vi "OG_HTML_String.vi"(11 "Cluster":T1) -> (3 "String":string)   [LabVIEW 2018]
uses:
  MainFrame/TypeDefs/InternalDataCluster.ctl
  Private Controls/Report Data Cluster.ctl
  Private Controls/Data Raw.ctl
  Data Operations.lvlib
  MainFrame/MainFrameLib.lvlib
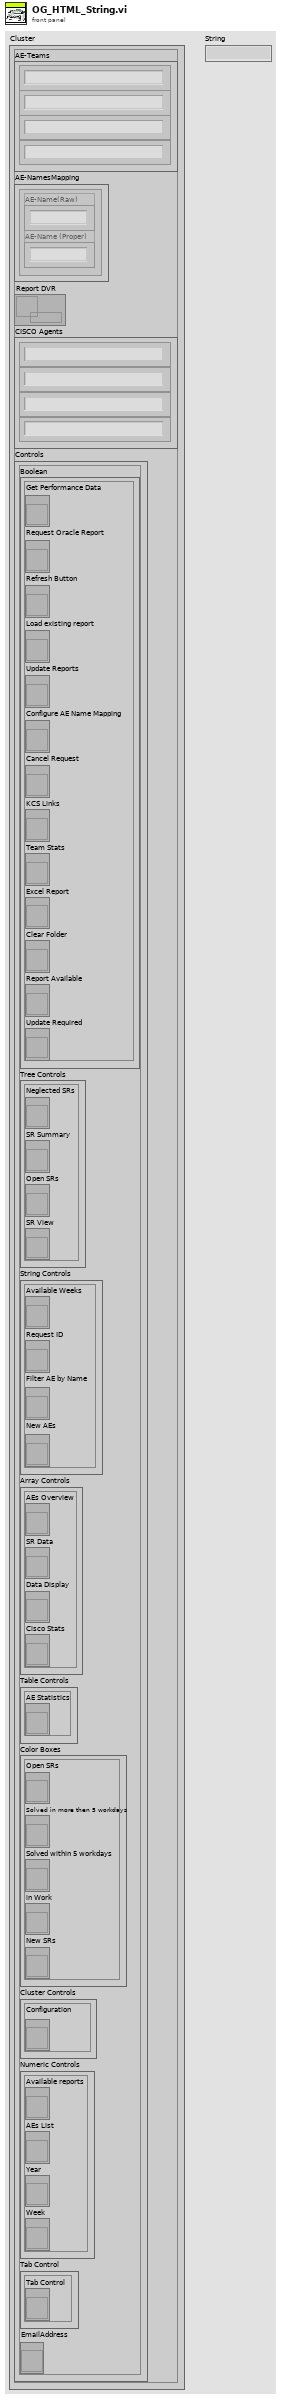
[diagram p1: front panel]
types:
  T1 = typedef "MainFrameLib.lvlib/InternalDataCluster.ctl" = cluster{"AE-Teams":string[], "AE-NamesMapping":cluster{"AE-Name(Raw)":string, "AE-Name (Proper)":string}[], "Report DVR":refnum<data-value>, "CISCO Agents":string[], "Controls":cluster{"Boolean":cluster{"Get Performance Data":refnum<vi>, "Request Oracle Report":refnum<vi>, "Refresh Button":refnum<vi>, "Load existing report":refnum<vi>, "Update Reports":refnum<vi>, "Configure AE Name Mapping":refnum<vi>, "Cancel Request":refnum<vi>, "KCS Links":refnum<vi>, "Team Stats":refnum<vi>, "Excel Report":refnum<vi>, "Clear Folder":refnum<vi>, "Report Available":refnum<vi>, "Update Required":refnum<vi>}, "Tree Controls":cluster{"Neglected SRs":refnum<vi>, "SR Summary":refnum<vi>, "Open SRs":refnum<vi>, "SR View":refnum<vi>}, "String Controls":cluster{"Available Weeks":refnum<vi>, "Request ID":refnum<vi>, "Filter AE by Name":refnum<vi>, "New AEs":refnum<vi>}, "Array Controls":cluster{"AEs Overview":refnum<vi>, "SR Data":refnum<vi>, "Data Display":refnum<vi>, "Cisco Stats":refnum<vi>}, "Table Controls":cluster{"AE Statistics":refnum<vi>}, "Color Boxes":cluster{"Open SRs":refnum<vi>, "Solved in more then 5 workdays":refnum<vi>, "Solved within 5 workdays":refnum<vi>, "in Work":refnum<vi>, "New SRs":refnum<vi>}, "Cluster Controls":cluster{"Configuration":refnum<vi>}, "Numeric Controls":cluster{"Available reports":refnum<vi>, "AEs List":refnum<vi>, "Year":refnum<vi>, "Week":refnum<vi>}, "Tab Control":cluster{"Tab Control":refnum<vi>}, "EmailAddress":refnum<vi>}}
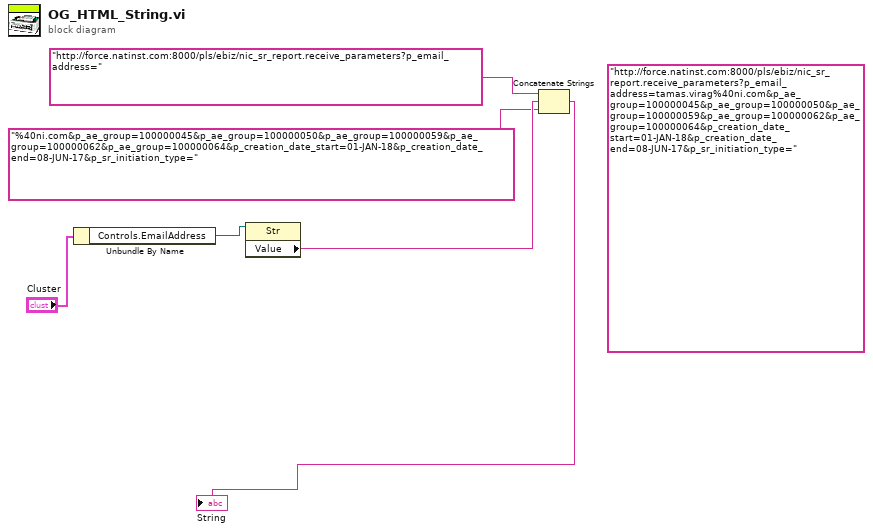
[diagram p0: block diagram]
diagram:
  (unwired) "http://force.natinst.com:8000/pls/ebiz/nic_sr_report.receive_parameters?p_email_address=tamas.virag%40ni.com&p_ae_group=100000045&p_ae_group=100000050&p_ae_group=100000059&p_ae_group=100000062&p_ae_group=100000064&p_creation_date_start=01-JAN-18&p_creation_date_end=08-JUN-17&p_sr_initiation_type=" ("HTTP string")
  n1 = Unbundle By Name("Cluster") -> ("Controls.EmailAddress"=w2:refnum<vi>)
  n2 = property class="Str"(reference=w2) -> ("Value"=w5:string)  [unwired: 1 in, 2 out]
  n3 = Concatenate Strings("http://force.natinst.com:8000/pls/ebiz/nic_sr_report.receive_parameters?p_email_address=" ("string"), w5, "%40ni.com&p_ae_group=100000045&p_ae_group=100000050&p_ae_group=100000059&p_ae_group=100000062&p_ae_group=100000064&p_creation_date_start=01-JAN-18&p_creation_date_end=08-JUN-17&p_sr_initiation_type=" ("string")) -> (→"String":string)
